vi "DeferPanelUpdate.vi"(8 "error in (no error)":errorcluster, 10 "Defer Panel Updates":bool, 11 "VI in":refnum<vi>) -> (0 "error out":errorcluster)   [LabVIEW 2016, in "EmbeddedSMO.lvclass"]
uses:
  EmbeddedSMO.lvclass
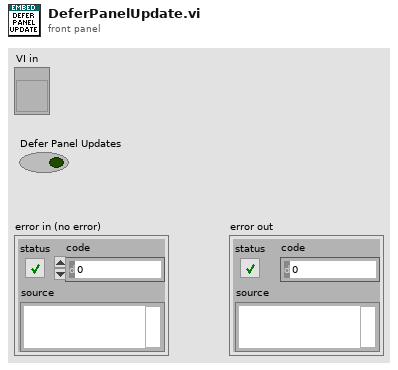
[diagram p1: front panel]
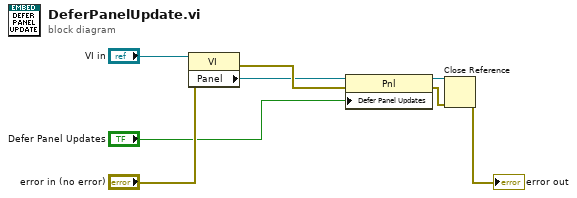
[diagram p0: block diagram]
diagram:
  n1 = property class="VI"(reference="VI in", error in="error in (no error)") -> (error out=w8:errorcluster, "Panel"=w7:refnum<vi>)  [unwired: 1 out]
  n2 = property class="Pnl"(reference=w7, error in=w8, "Defer Panel Updates"="Defer Panel Updates") -> (reference out=w3:refnum<vi>, error out=w1:errorcluster)
  n3 = Close Reference(reference=w3, error in (no error)=w1) -> (error out=→"error out":errorcluster)
